vi "GUI_Magspec_BELLA_oldschool.vi"() -> ()   [LabVIEW 2013]
uses:
  shared programs/GUI_Template/GUI_master/tcp_new_data_event.ctl
  shared programs/GUI_Template/GUI_master/tcp new data cluster.ctl
  shared programs/MySQL/Preset Query Enum.ctl
  <vilib>/Analysis/2dsp.llb/Decimate (single shot, DBL).vi
  <vilib>/Utility/tcp.llb/UDP Multicast Read-Only Open.vi
  <vilib>/Analysis/NI_AALPro.lvlib
  <vilib>/vision/NI_Vision_Development_Module.lvlib
panel:
  in  "multiplier":sgl=1.0 format="%.2f"
  out "ImageInterp::3":T1(plugin-control) caption="C cam"
  out "ShotNumber":i32
  out "data":string[][](array[string])
  out "error out 3":errorcluster
  out "image::13":T1(plugin-control) caption="Beam Profile"
  in  "rank for LPF":i32=2
  out "Momentum 25":dbl=2.780793 caption="Momentum (GeV/c)" min=0.0 max=0.0 format="%#.1f"
  out "Momentum 24":dbl=2.780793 caption="Momentum (GeV/c)" min=0.0 max=0.0 format="%#.1f"
  out "Momentum 23":dbl=2.780793 caption="Momentum (GeV/c)" min=0.0 max=0.0 format="%#.1f"
  out "Momentum 22":dbl=2.780793 caption="Momentum (GeV/c)" min=0.0 max=0.0 format="%#.1f"
  out "Momentum 21":dbl=2.780793 caption="Momentum (GeV/c)" min=0.0 max=0.0 format="%#.1f"
  out "Momentum 20":dbl=2.780793 caption="Momentum (GeV/c)" min=0.0 max=0.0 format="%#.1f"
  out "Momentum 19":dbl=2.780793 caption="Momentum (GeV/c)" min=0.0 max=0.0 format="%#.1f"
  out "Momentum 18":dbl=2.780793 caption="Momentum (GeV/c)" min=0.0 max=0.0 format="%#.1f"
  out "Momentum 17":dbl=2.780793 caption="Momentum (GeV/c)" min=0.0 max=0.0 format="%#.1f"
  out "Momentum 16":dbl=2.780793 caption="Momentum (GeV/c)" min=0.0 max=0.0 format="%#.1f"
  out "Momentum 15":dbl=2.780793 caption="Momentum (GeV/c)" min=0.0 max=0.0 format="%#.1f"
  out "Waveform Graph":dbl[](graph)
  in  "HorizontalLineout::12":dbl[](array[numeric]) caption="HorizontalLineout MagSpecA"
  in  "HorizontalLineout::11":dbl[](array[numeric]) caption="HorizontalLineout MagSpecA"
  in  "HorizontalLineout::10":dbl[](array[numeric]) caption="HorizontalLineout MagSpecA"
  in  "HorizontalLineout::9":dbl[](array[numeric]) caption="HorizontalLineout MagSpecA"
  in  "HorizontalLineout::8":dbl[](array[numeric]) caption="HorizontalLineout MagSpecA"
  in  "HorizontalLineout::7":dbl[](array[numeric]) caption="HorizontalLineout MagSpecA"
  in  "HorizontalLineout::6":dbl[](array[numeric]) caption="HorizontalLineout MagSpecA"
  in  "HorizontalLineout::5":dbl[](array[numeric]) caption="HorizontalLineout MagSpecA"
  in  "HorizontalLineout::4":dbl[](array[numeric]) caption="HorizontalLineout MagSpecA"
  in  "HorizontalLineout::3":dbl[](array[numeric]) caption="HorizontalLineout MagSpecA"
  in  "HorizontalLineout::2":dbl[](array[numeric]) caption="HorizontalLineout MagSpecA"
  in  "HorizontalLineout::1":dbl[](array[numeric]) caption="HorizontalLineout MagSpecA"
  out "error out 2":errorcluster
  out "error out":errorcluster
  out "Momentum 14":dbl=2.780793 caption="Momentum (GeV/c)" min=0.0 max=0.0 format="%#.1f"
  out "Momentum 13":dbl=2.780793 caption="Momentum (GeV/c)" min=0.0 max=0.0 format="%#.1f"
  out "Momentum 12":dbl=2.780793 caption="Momentum (GeV/c)" min=0.0 max=0.0 format="%#.1f"
  out "Momentum 11":dbl=2.780793 caption="Momentum (GeV/c)" min=0.0 max=0.0 format="%#.1f"
  out "Momentum 10":dbl=2.780793 caption="Momentum (GeV/c)" min=0.0 max=0.0 format="%#.1f"
  out "Momentum 9":dbl=2.780793 caption="Momentum (GeV/c)" min=0.0 max=0.0 format="%#.1f"
  out "Momentum 8":dbl=2.780793 caption="Momentum (GeV/c)" min=0.0 max=0.0 format="%#.1f"
  out "Momentum 7":dbl=2.780793 caption="Momentum (GeV/c)" min=0.0 max=0.0 format="%#.1f"
  out "Momentum 6":dbl=2.780793 caption="Momentum (GeV/c)" min=0.0 max=0.0 format="%#.1f"
  out "Momentum 5":dbl=2.780793 caption="Momentum (GeV/c)" min=0.0 max=0.0 format="%#.1f"
  out "Momentum 4":dbl=2.780793 caption="Momentum (GeV/c)" min=0.0 max=0.0 format="%#.1f"
  out "Momentum 3":dbl=2.780793 caption="Momentum (GeV/c)" min=0.0 max=0.0 format="%#.1f"
  out "Momentum 2":dbl=2.780793 caption="Momentum (GeV/c)" min=0.0 max=0.0 format="%#.1f"
  out "Momentum 1":dbl=2.780793 caption="Momentum (GeV/c)" min=0.0 max=0.0 format="%#.1f"
  in  "GUIdevice 14":string="BELLA_HallProbe"
  out "EBeamFlp":T1(plugin-control) caption="Beam Profile"
  out "image::12":T1(plugin-control) caption="L Cam"
  out "image::11":T1(plugin-control) caption="K Cam"
  out "image::10":T1(plugin-control) caption="J Cam"
  out "image::9":T1(plugin-control) caption="I Cam"
  in  "GUIdevice 12":string="MagSpecL"
  in  "GUIdevice 11":string="MagSpecK"
  in  "GUIdevice 10":string="MagSpecJ"
  in  "GUIdevice 9":string="MagSpecI"
  in  "GUIdevice 8":string="MagSpecH"
  out "image::8":T1(plugin-control) caption="H Cam"
  in  "GUIdevice 7":string="MagSpecG"
  in  "GUIdevice 6":string="MagSpecF"
  out "image::7":T1(plugin-control) caption="G Cam"
  out "image::6":T1(plugin-control) caption="F Cam"
  in  "GUIdevice 5":string="MagSpecE"
  out "image::5":T1(plugin-control) caption="E Cam"
  out "flipped2":T1(plugin-control) caption="M1 Cam"
  out "flipped1":T1(plugin-control) caption="A Cam"
  out "image::4":T1(plugin-control) caption="D Cam"
  out "image::3":T1(plugin-control) caption="C cam"
  out "image::2":T1(plugin-control) caption="B Cam"
  in  "GUIdevice 4":string="MagSpecD"
  in  "GUIdevice 3":string="MagSpecC"
  in  "GUIdevice 2":string="MagSpecB"
  out "image::1":T1(plugin-control) caption="A Cam"
  in  "Field::14":dbl=2.780793 caption="Magnetic Field (mT)" min=0.0 max=0.0 format="%_4f"
  in  "GUIdevice 13":string="EBeam_Profile_BELLA_1"
  in  "GUIdevice 1":string="MagSpecA"
  out "tcp data event":T2
  in  "stop":bool
  out "error IO 2":errorcluster
  out "Boolean":bool
  # "AA side"
  # "T\no\np"
  # "B\nT\nM"
  # "Parking side"
  # "Beam Axis"
  # "MeV/c"
  # "MeV/c"
  # "MeV/c"
  # "MeV/c"
  # "MeV/c"
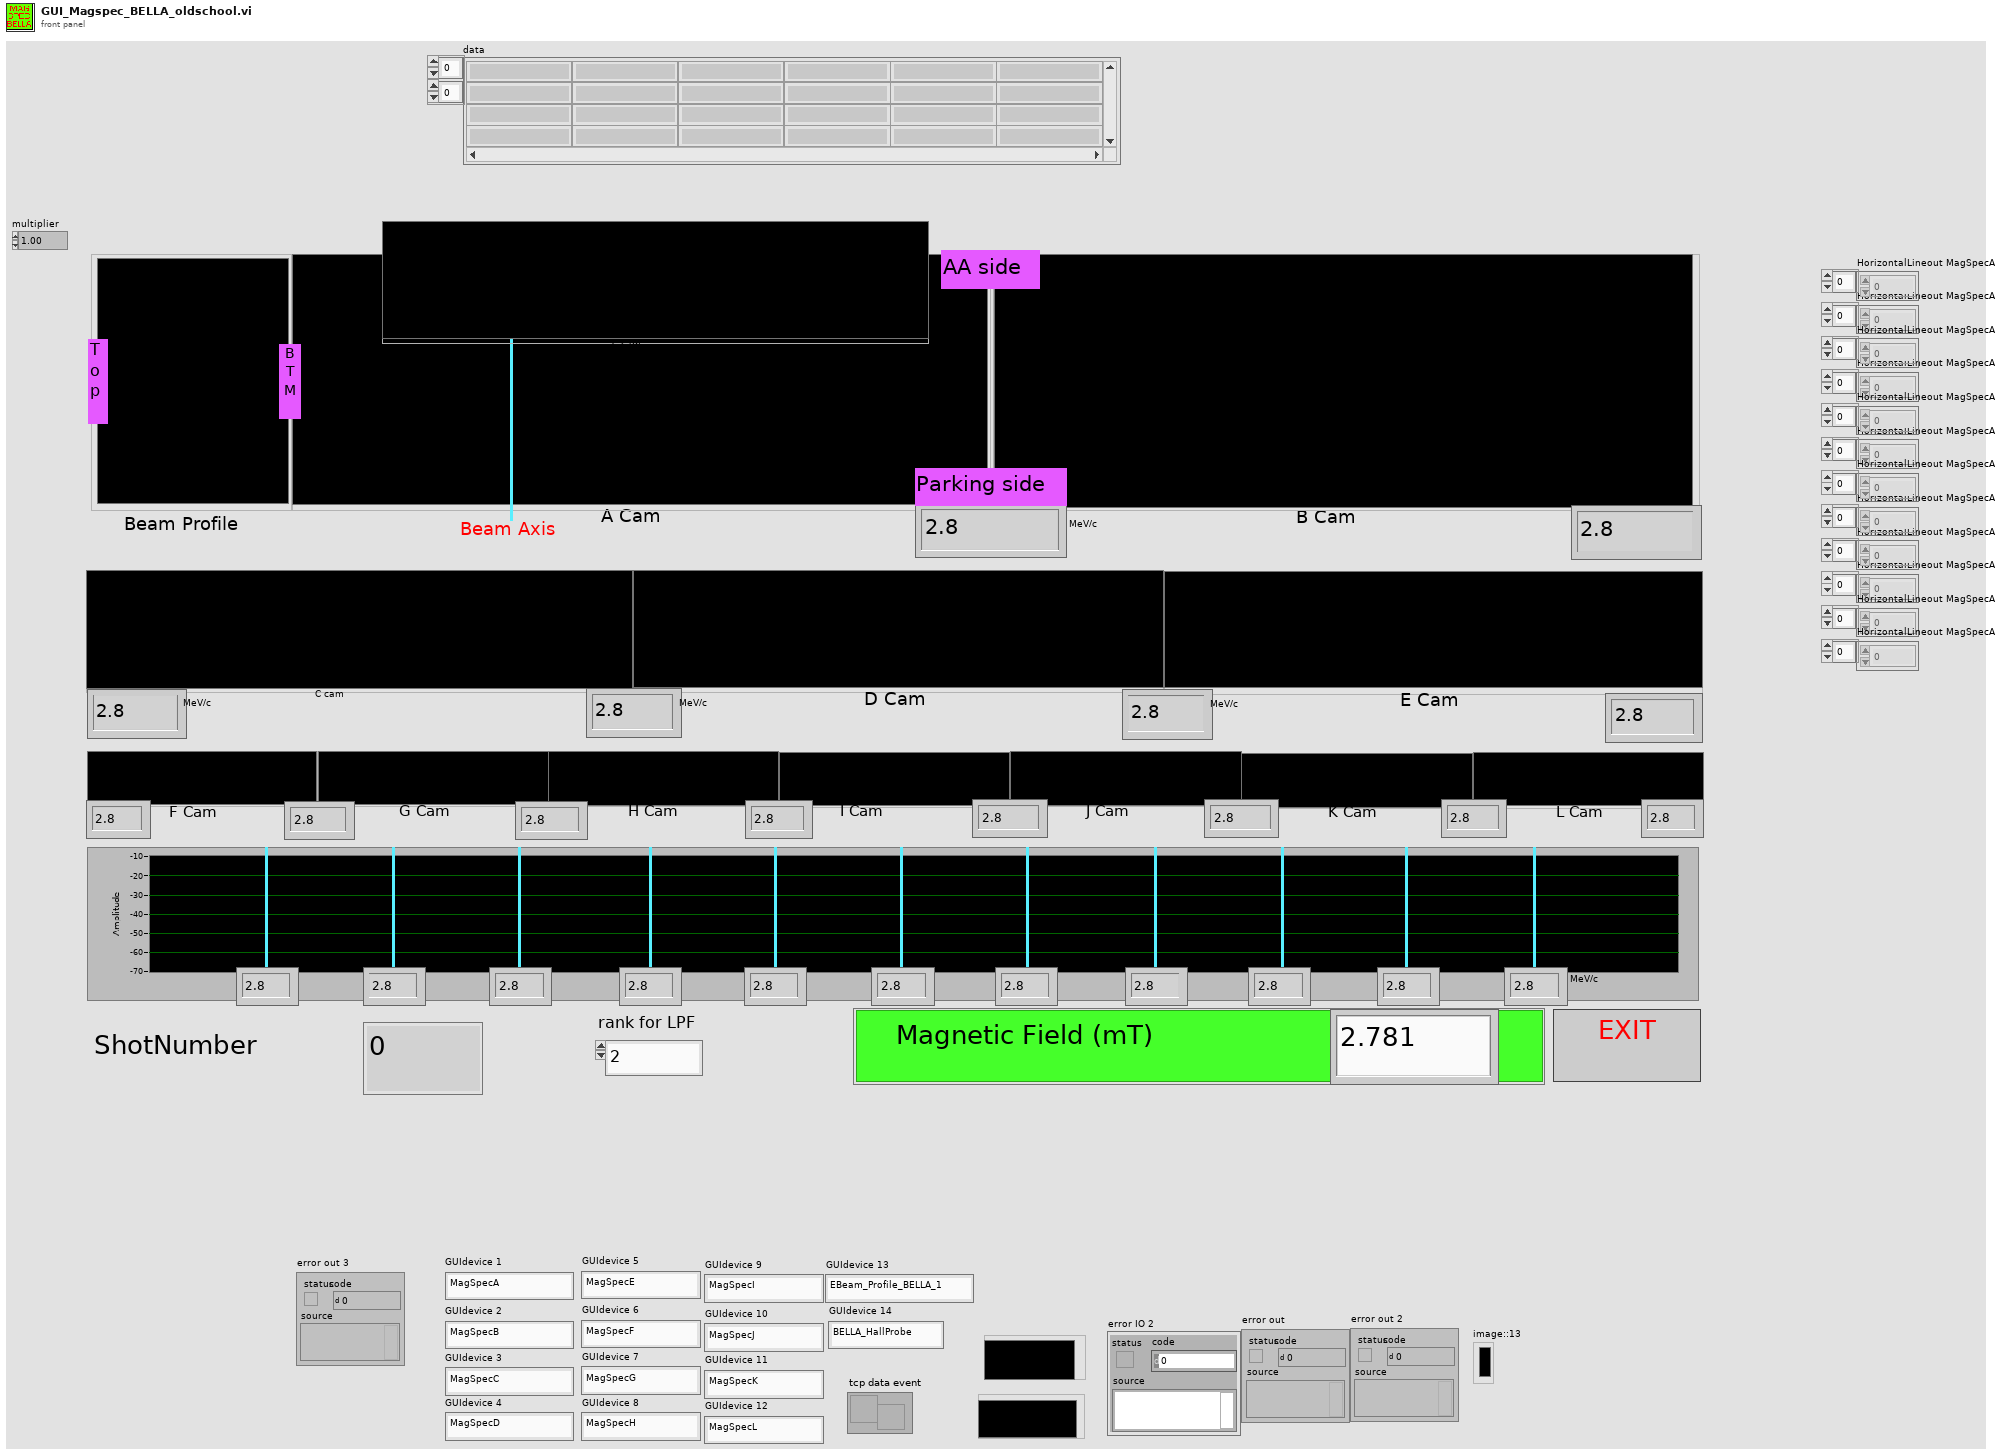
[diagram p1: front panel]
types:
  T1 = typedef "IMAQ Image.ctl" = refnum<image>
  T2 = typedef "tcp_new_data_event.ctl" = refnum<user-event>
  T3 = typedef "Image Type" = u32
  T4 = typedef "Preset Query Enum.ctl" = enum16{"Get Locations", "Get all IPs and MACs", "Get classes", "Get expt variables to set at scanstart for particular device", "Get expt devices and variables with start values", "Get expt devices and variables (with data to get)", "Get expt devices with data to get", "Get Expt devices and GUIs", "Get all devices basic properties", "Get Virtual Devices Core Info", "Get Expt names", "Get experiment basic properties", "Get experiment alarm variables", "Get MC Ports", "Get device network comm port", "Get devicetype lvclass path", "Get basic device properties", "Get Init Order", "Get all setable variables of a device", "Get device variable aliases", "Get force values of all settable variables", "Get all variables of a devicetype", "Get all variables of a device", "Get plotter details", "Get Saved Scans", "Get Scan Info", "GetGeneralGUIs", "Get expt for plotter", "Get plotter IDs from expt", "Get all devices", "Get all Virtual Devices", "Get all aliases", "Get variable and device info for Virtual Device", "GetItemLocatorIP", "Get IPs for GUIs", "Get DeviceType from Device", "GetLocalPortRange", "GetDevicePresetVariables", "Get Device Configuration", "GetAllPresetNames", "GetAllConfigurationNames", "GetPresetDeviceNames"}
  T5 = typedef "tcp new data cluster.ctl" = cluster{"EventEnum":enum16{"new data", "connection status update"}, "Device name":string}
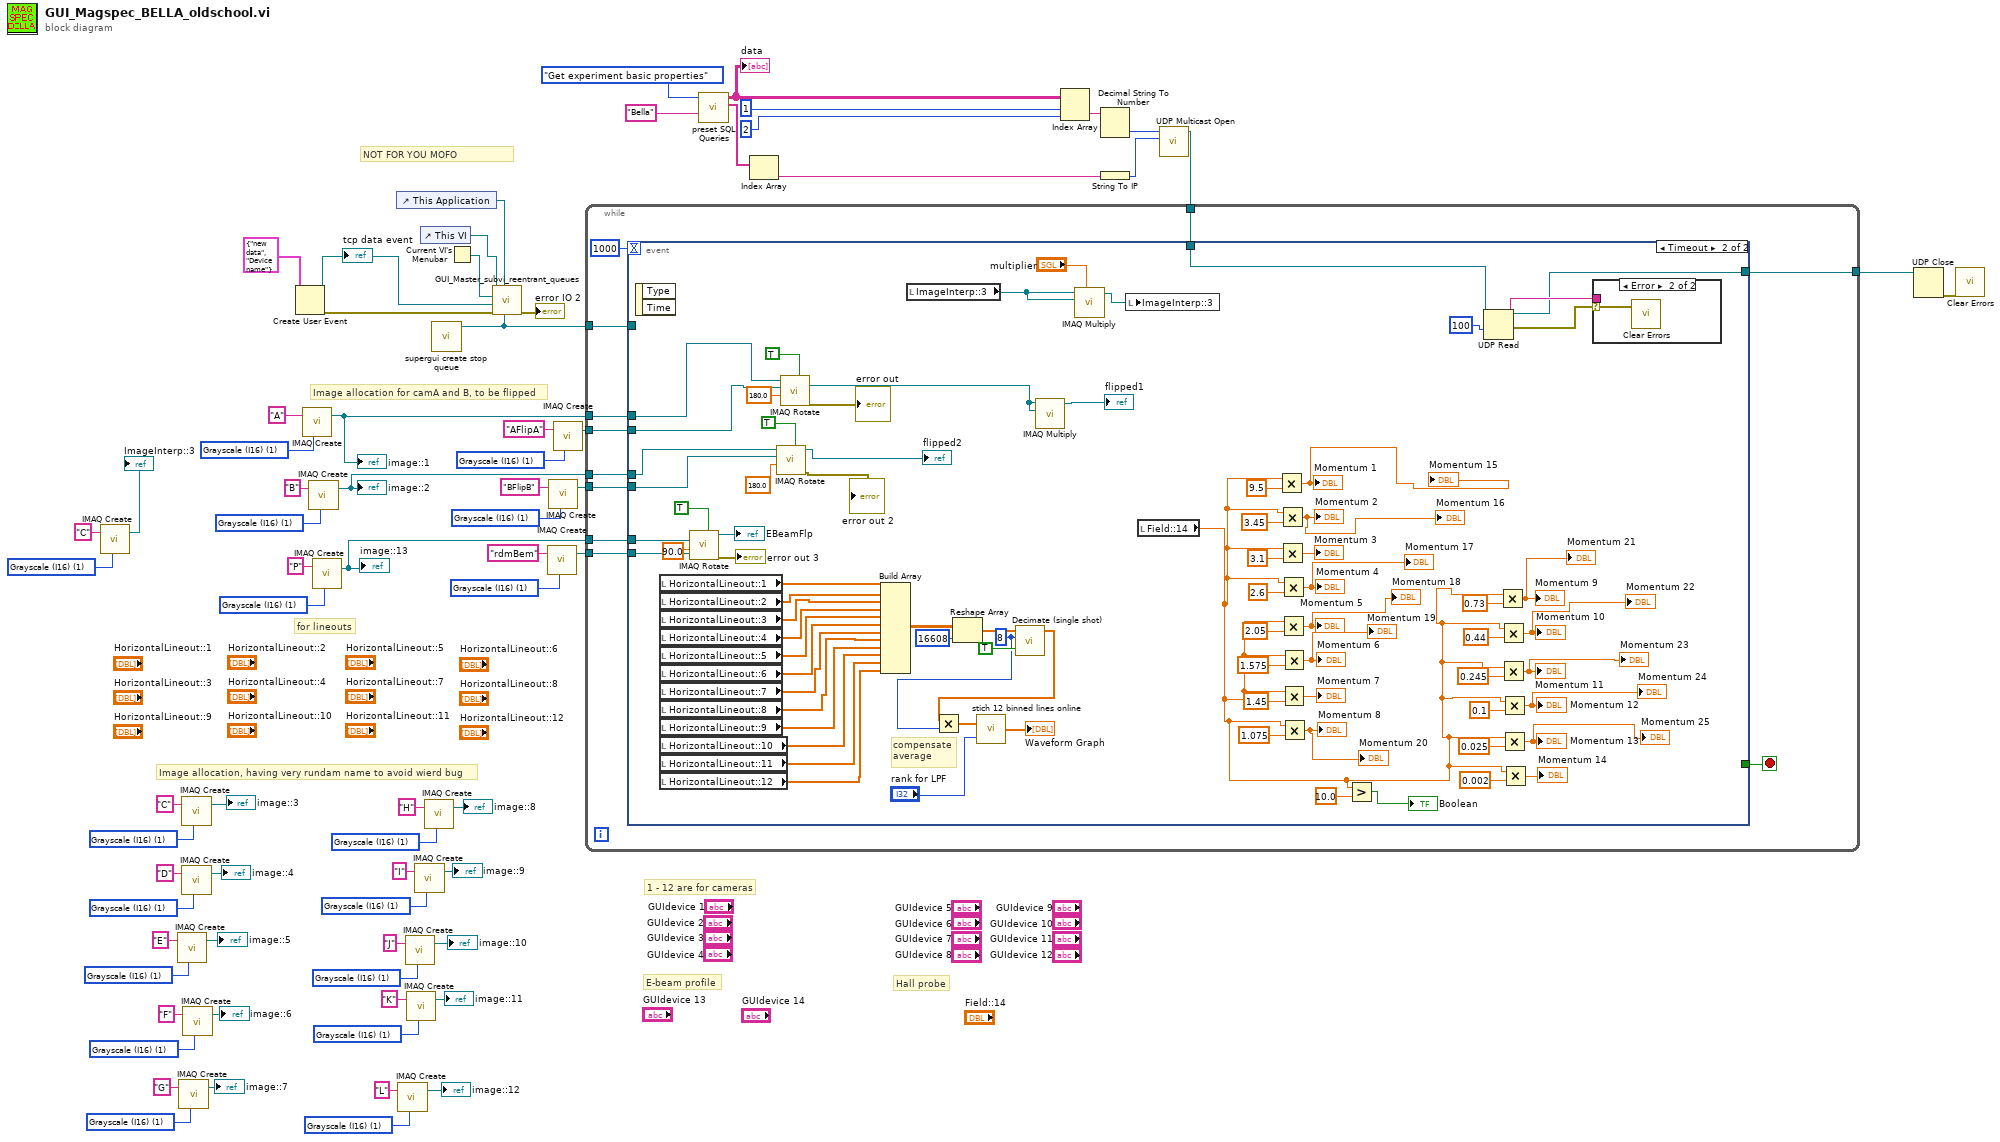
[diagram p0: block diagram]
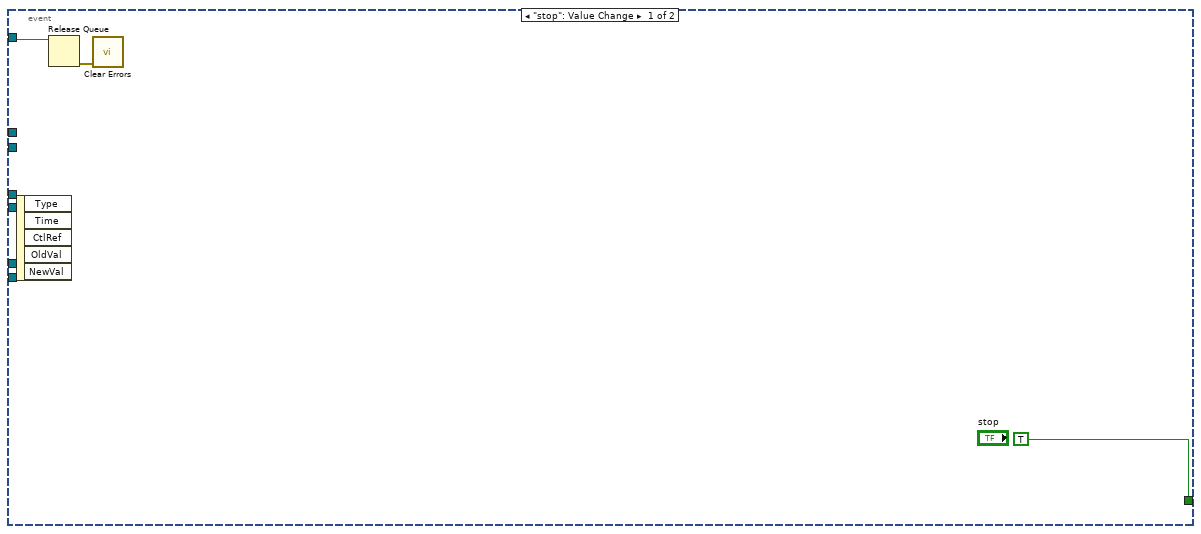
[diagram p2: hidden frame]
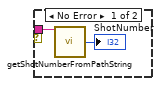
[diagram p3: hidden frame]
diagram:
  w1 = T3 1 items=["Grayscale (U8)", "Grayscale (I16)", "Grayscale (SGL)", "Complex (CSG)", "RGB (U32)", "HSL (U32)", "RGB (U64)", "Grayscale (U16)"] ("Image Type")
  w20 = T3 1 items=["Grayscale (U8)", "Grayscale (I16)", "Grayscale (SGL)", "Complex (CSG)", "RGB (U32)", "HSL (U32)", "RGB (U64)", "Grayscale (U16)"] ("Image Type")
  w35 = T3 1 items=["Grayscale (U8)", "Grayscale (I16)", "Grayscale (SGL)", "Complex (CSG)", "RGB (U32)", "HSL (U32)", "RGB (U64)", "Grayscale (U16)"] ("Image Type")
  w36 = T3 1 items=["Grayscale (U8)", "Grayscale (I16)", "Grayscale (SGL)", "Complex (CSG)", "RGB (U32)", "HSL (U32)", "RGB (U64)", "Grayscale (U16)"] ("Image Type")
  w39 = T3 1 items=["Grayscale (U8)", "Grayscale (I16)", "Grayscale (SGL)", "Complex (CSG)", "RGB (U32)", "HSL (U32)", "RGB (U64)", "Grayscale (U16)"] ("Image Type")
  w40 = T3 1 items=["Grayscale (U8)", "Grayscale (I16)", "Grayscale (SGL)", "Complex (CSG)", "RGB (U32)", "HSL (U32)", "RGB (U64)", "Grayscale (U16)"] ("Image Type")
  w43 = T3 1 items=["Grayscale (U8)", "Grayscale (I16)", "Grayscale (SGL)", "Complex (CSG)", "RGB (U32)", "HSL (U32)", "RGB (U64)", "Grayscale (U16)"] ("Image Type")
  w44 = T3 1 items=["Grayscale (U8)", "Grayscale (I16)", "Grayscale (SGL)", "Complex (CSG)", "RGB (U32)", "HSL (U32)", "RGB (U64)", "Grayscale (U16)"] ("Image Type")
  w47 = T3 1 items=["Grayscale (U8)", "Grayscale (I16)", "Grayscale (SGL)", "Complex (CSG)", "RGB (U32)", "HSL (U32)", "RGB (U64)", "Grayscale (U16)"] ("Image Type")
  w48 = T3 1 items=["Grayscale (U8)", "Grayscale (I16)", "Grayscale (SGL)", "Complex (CSG)", "RGB (U32)", "HSL (U32)", "RGB (U64)", "Grayscale (U16)"] ("Image Type")
  w51 = T3 1 items=["Grayscale (U8)", "Grayscale (I16)", "Grayscale (SGL)", "Complex (CSG)", "RGB (U32)", "HSL (U32)", "RGB (U64)", "Grayscale (U16)"] ("Image Type")
  w52 = T3 1 items=["Grayscale (U8)", "Grayscale (I16)", "Grayscale (SGL)", "Complex (CSG)", "RGB (U32)", "HSL (U32)", "RGB (U64)", "Grayscale (U16)"] ("Image Type")
  w55 = T3 1 items=["Grayscale (U8)", "Grayscale (I16)", "Grayscale (SGL)", "Complex (CSG)", "RGB (U32)", "HSL (U32)", "RGB (U64)", "Grayscale (U16)"] ("Image Type")
  w56 = T3 1 items=["Grayscale (U8)", "Grayscale (I16)", "Grayscale (SGL)", "Complex (CSG)", "RGB (U32)", "HSL (U32)", "RGB (U64)", "Grayscale (U16)"] ("Image Type")
  w59 = T3 1 items=["Grayscale (U8)", "Grayscale (I16)", "Grayscale (SGL)", "Complex (CSG)", "RGB (U32)", "HSL (U32)", "RGB (U64)", "Grayscale (U16)"] ("Image Type")
  w62 = T3 1 items=["Grayscale (U8)", "Grayscale (I16)", "Grayscale (SGL)", "Complex (CSG)", "RGB (U32)", "HSL (U32)", "RGB (U64)", "Grayscale (U16)"] ("Image Type")
  w63 = T3 1 items=["Grayscale (U8)", "Grayscale (I16)", "Grayscale (SGL)", "Complex (CSG)", "RGB (U32)", "HSL (U32)", "RGB (U64)", "Grayscale (U16)"] ("Image Type")
  # "for lineouts"
  # "Hall probe"
  # "E-beam profile"
  # "1 - 12 are for cameras"
  # "Image allocation for camA and B, to be flipped"
  # "Image allocation, having very rundam name to avoid wierd bug"
  # "NOT FOR YOU MOFO"
  n1 = call "IMAQ Create"("Image Name"="C", "Image Type"=w1) -> ("New Image"=→"ImageInterp::3":T1)  [unwired: 3 in, 1 out]
  n2 = call "IMAQ Create"("Image Name"="E", "Image Type"=w51) -> ("New Image"=→"image::5":T1)  [unwired: 3 in, 1 out]
  n3 = call "IMAQ Create"("Image Name"="G", "Image Type"=w47) -> ("New Image"=→"image::7":T1)  [unwired: 3 in, 1 out]
  n4 = call "IMAQ Create"("Image Name"="C", "Image Type"=w55) -> ("New Image"=→"image::3":T1)  [unwired: 3 in, 1 out]
  n5 = call "IMAQ Create"("Image Name"="D", "Image Type"=w52) -> ("New Image"=→"image::4":T1)  [unwired: 3 in, 1 out]
  n6 = call "IMAQ Create"("Image Name"="F", "Image Type"=w48) -> ("New Image"=→"image::6":T1)  [unwired: 3 in, 1 out]
  n7 = Create User Event(user event datatype=T5 {"EventEnum"=enum."new data", "Device name"="Device name"} ("New Event")) -> (user event=w71:refnum<user-event>, error out=w70:errorcluster)  [unwired: 1 in]
  "tcp data event" <- w71
  n8 = call "IMAQ Create"("Image Name"="A", "Image Type"=w59) -> ("New Image"=w33:T1)  [unwired: 3 in, 1 out]
  "image::1" <- w33
  n9 = call "IMAQ Create"("Image Name"="B", "Image Type"=w56) -> ("New Image"=w32:T1)  [unwired: 3 in, 1 out]
  "image::2" <- w32
  n10 = call "IMAQ Create"("Image Name"="P", "Image Type"=w35) -> ("New Image"=w18:T1)  [unwired: 3 in, 1 out]
  "image::13" <- w18
  n11 = control-ref of="This Application"() -> (w72:refnum<vi>)
  n12 = call "IMAQ Create"("Image Name"="L", "Image Type"=w36) -> ("New Image"=→"image::12":T1)  [unwired: 3 in, 1 out]
  n13 = call "IMAQ Create"("Image Name"="J", "Image Type"=w40) -> ("New Image"=→"image::10":T1)  [unwired: 3 in, 1 out]
  n14 = call "IMAQ Create"("Image Name"="K", "Image Type"=w39) -> ("New Image"=→"image::11":T1)  [unwired: 3 in, 1 out]
  n15 = call "IMAQ Create"("Image Name"="I", "Image Type"=w43) -> ("New Image"=→"image::9":T1)  [unwired: 3 in, 1 out]
  n16 = control-ref of="This VI"() -> (w67:refnum<vi>)
  n17 = call "IMAQ Create"("Image Name"="H", "Image Type"=w44) -> ("New Image"=→"image::8":T1)  [unwired: 3 in, 1 out]
  n18 = call "supergui create stop queue.vi"() -> ("STOP Queue out"=w4:refnum<queue>)  [unwired: 11 in]
  n19 = Current VI's Menubar() -> (w68:refnum<k9>)
  n20 = call "GUI_Master_subvi_reentrant_queues.vi"("STOP Queue in"=w4, "This Application"=w72, "error in (no error)"=w70, "tcp data event"=w71, "Caller menu reference"=w68, "Caller VI ref"=w67) -> ("error out"=→"error IO 2":errorcluster)  [unwired: 5 in]
  n21 = call "IMAQ Create"("Image Name"="rdmBem", "Image Type"=w20) -> ("New Image"=w19:T1)  [unwired: 3 in, 1 out]
  n22 = call "IMAQ Create"("Image Name"="BFlipB", "Image Type"=w62) -> ("New Image"=w60:T1)  [unwired: 3 in, 1 out]
  n23 = call "IMAQ Create"("Image Name"="AFlipA", "Image Type"=w63) -> ("New Image"=w64:T1)  [unwired: 3 in, 1 out]
  n24 = call "preset SQL Queries.vi"("Expt name / MCIP/ Variable/Preset Name"="Bella", "Preset Query"=Preset_Query_Enum."Get experiment basic properties") -> ("1st column 1st data"=w10:string[], "data"=w11:string[][])  [unwired: 7 in, 1 out]
  "data" <- w11
  n25 = Index Array(array=w10) -> (element=w9:string)  [unwired: 1 in]
  n26 = Index Array(array=w11, index (row)=1, index (col)=2 ("disabled index (col)")) -> (element=w12:string)
  n27 = Decimal String To Number(string=w12) -> (number=w8:i32)  [unwired: 2 in, 1 out]
  n28 = String To IP(1:w9) -> (0:w15:u32)
  n29 = call-poly <vilib>:"UDP Multicast Open.vi"("multicast addr"=w15, "port"=w8) -> ("connection ID"=w7:refnum<k16>)  [unwired: 7 in, 2 out]
  n30 = while {
    tunnel: w33 -> [w82]
    tunnel: w64 -> [w81]
    tunnel: w60 -> [w80]
    tunnel: w32 -> [w79]
    tunnel: w18 -> [w78]
    tunnel: w19 -> [w77]
    tunnel: w7 -> [w76]
    tunnel: [w75] -> w6
    tunnel: w4 -> [w73]
    stop <- w83 stop-if-true
    n31 = event shown="[1] Timeout" {
      selector: _ -> [_ _]
      dyn-events: _ -> [_ _]
      timeout: 1000 -> [_ _]
      tunnel: [TRUE ("stop") _] -> w83
      tunnel: w82 -> [_ w98]
      tunnel: w81 -> [_ w97]
      tunnel: w80 -> [_ w154]
      tunnel: w79 -> [_ w155]
      tunnel: w78 -> [_ w161]
      tunnel: w77 -> [_ w160]
      tunnel: w76 -> [_ w93]
      tunnel: [_ w92] -> w75
      tunnel: w73 -> [w85 _]
      event "stop": Value Change {
        n32 = event-data() -> ()  [unwired: 1 in, 5 out]
        n33 = Release Queue(queue=w85) -> (error out=w84:errorcluster)  [unwired: 2 in, 2 out]
        n34 = call <vilib>:"Clear Errors.vi"("error in (no error)"=w84) -> ()  [unwired: 6 in, 1 out]
      }
      event Timeout {
        w103 = 8 ("decimating factor")
        # "compensate\naverage"
        n35 = event-data() -> ()  [unwired: 1 in, 2 out]
        n36 = local read "HorizontalLineout::1"() -> (w122:dbl[])
        n37 = local read "HorizontalLineout::2"() -> (w121:dbl[])
        n38 = local read "HorizontalLineout::3"() -> (w120:dbl[])
        n39 = local read "HorizontalLineout::4"() -> (w119:dbl[])
        n40 = local read "HorizontalLineout::5"() -> (w118:dbl[])
        n41 = local read "HorizontalLineout::6"() -> (w117:dbl[])
        n42 = local read "HorizontalLineout::7"() -> (w116:dbl[])
        n43 = local read "HorizontalLineout::8"() -> (w115:dbl[])
        n44 = local read "HorizontalLineout::9"() -> (w114:dbl[])
        n45 = local read "HorizontalLineout::10"() -> (w113:dbl[])
        n46 = local read "HorizontalLineout::11"() -> (w112:dbl[])
        n47 = local read "HorizontalLineout::12"() -> (w111:dbl[])
        n48 = call "IMAQ Rotate"("Maintain Size"=TRUE, "Angle (degrees)"=sgl 90.0, "Image Dst"=w160, "Image Src"=w161) -> ("error out"=→"error out 3":errorcluster, "Image Dst Out"=→"EBeamFlp":T1)  [unwired: 6 in]
        n49 = call "IMAQ Rotate"("Maintain Size"=TRUE, "Angle (degrees)"=sgl 180.0, "Image Dst"=w154, "Image Src"=w155) -> ("error out"=→"error out 2":errorcluster, "Image Dst Out"=→"flipped2":T1)  [unwired: 6 in]
        n50 = call "IMAQ Rotate"("Maintain Size"=TRUE, "Angle (degrees)"=sgl 180.0, "Image Dst"=w97, "Image Src"=w98) -> ("error out"=→"error out":errorcluster, "Image Dst Out"=w89:T1)  [unwired: 6 in]
        n51 = Build Array(w122, w121, w120, w119, w118, w117, w116, w115, w114, w113, w112, w111) -> (w110:dbl[][])
        n52 = local read "ImageInterp::3"() -> (w91:T1)
        n53 = Reshape Array(w110, 16608 ("dimension size")) -> (w108:dbl[])
        n54 = call-poly <vilib>:"Decimate (single shot).vi"("averaging"=TRUE, "decimating factor"=w103, "X"=w108) -> ("Decimated Array"=w104:dbl[])  [unwired: 7 in, 1 out]
        n55 = Multiply(x=w104, y=w103) -> (x*y=w105:dbl[])
        n56 = call "stich 12 binned lines online.vi"("rank"="rank for LPF", "Input"=w105) -> ("stiched signal"=→"Waveform Graph":dbl[])
        n57 = call "IMAQ Multiply"("Image Src A"=w89, "Image Dst"=w89) -> ("Image Dst Out"=→"flipped1":T1)  [unwired: 5 in, 1 out]
        n58 = call "IMAQ Multiply"("Image Src A"=w91, "Constant"="multiplier", "Image Dst"=w91) -> ("Image Dst Out"=w87:T1)  [unwired: 4 in, 1 out]
        n59 = local write "ImageInterp::3"(w87) -> ()
        n60 = local read "Field::14"() -> (w153:dbl)
        n61 = Multiply(x=w153, y=9.5) -> (x*y=→"Momentum 1" →"Momentum 15":dbl)
        n62 = Multiply(x=w153, y=3.45) -> (x*y=→"Momentum 2" →"Momentum 16":dbl)
        n63 = Multiply(x=w153, y=3.1) -> (x*y=→"Momentum 3":dbl)
        n64 = Multiply(x=w153, y=2.6) -> (x*y=→"Momentum 4" →"Momentum 17":dbl)
        n65 = Multiply(x=w153, y=2.05) -> (x*y=→"Momentum 5" →"Momentum 18":dbl)
        n66 = Multiply(x=w153, y=1.575) -> (x*y=→"Momentum 6" →"Momentum 19":dbl)
        n67 = Multiply(x=w153, y=1.45) -> (x*y=→"Momentum 7":dbl)
        n68 = Multiply(x=w153, y=1.075) -> (x*y=→"Momentum 8" →"Momentum 20":dbl)
        n69 = Greater?(x=w153, y=10.0) -> (0:→"Boolean":bool)
        n70 = UDP Read(connection ID=w93, timeout ms (25000)=100) -> (data out=w95:string, error out=w94:errorcluster, 3:w92:refnum<k16>)  [unwired: 1 in, 3 out]
        n71 = Multiply(x=w153, y=0.73) -> (x*y=→"Momentum 9" →"Momentum 21":dbl)
        n72 = Multiply(x=w153, y=0.44) -> (x*y=→"Momentum 10" →"Momentum 22":dbl)
        n73 = Multiply(x=w153, y=0.245) -> (x*y=→"Momentum 11" →"Momentum 23":dbl)
        n74 = Multiply(x=w153, y=0.1) -> (x*y=→"Momentum 12" →"Momentum 24":dbl)
        n75 = Multiply(x=w153, y=0.025) -> (x*y=→"Momentum 13" →"Momentum 25":dbl)
        n76 = Multiply(x=w153, y=0.002) -> (x*y=→"Momentum 14":dbl)
        n77 = case shown="Error" w94 {
          selector: w94 -> [_ w168]
          tunnel: w95 -> [w167 _]
          frame No Error {
            n78 = call "getShotNumberFromPathString.vi"("Path String"=w167) -> ("ShotNumber from path"=→"ShotNumber":i32)
          }
          frame Error {
            n79 = call <vilib>:"Clear Errors.vi"("error in (no error)"=w168) -> ()  [unwired: 6 in, 1 out]
          }
        }
      }
    }
  }
  n80 = UDP Close(connection ID=w6) -> (error out=w5:errorcluster)  [unwired: 1 in, 1 out]
  n81 = call <vilib>:"Clear Errors.vi"("error in (no error)"=w5) -> ()  [unwired: 6 in, 1 out]
